vi "runtest empty test execution settings.vi"() -> (0 "empty Test Execution Settings":T1={"Quick Mode (T)"=FALSE, "Seq Count"=0, "Step Info"="", "Instruments on Station"=[], "LANGUAGE"="English", "Files Found?"=FALSE, "Step Number"=1} {"Step Number" min=1 step=1})   [LabVIEW 2011]
uses:
  tests/Test Execution Settings.ctl
  server/database/Stations/Instruments/Instrument Record.ctl
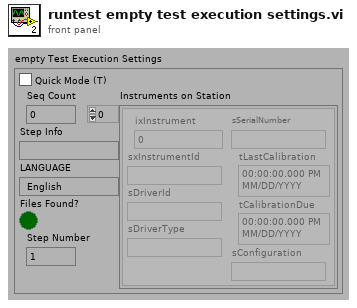
[diagram p1: front panel]
types:
  T1 = typedef "Test Execution Settings.ctl" = cluster{"Quick Mode (T)":bool, "Seq Count":i32, "Step Info":string, "Instruments on Station":T2[], "LANGUAGE":string, "Files Found?":bool, "Step Number":i32}
  T2 = typedef "Instrument Record.ctl" = cluster{"ixInstrument":i32, "sxInstrumentId":string, "sDriverId":string, "sDriverType":string, "sSerialNumber":string, "tLastCalibration":timestamp, "tCalibrationDue":timestamp, "sConfiguration":string}
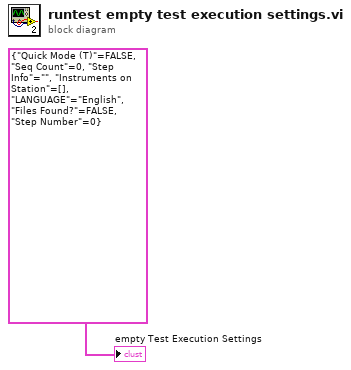
[diagram p0: block diagram]
diagram:
  "empty Test Execution Settings" <- T1 {"Quick Mode (T)"=FALSE, "Seq Count"=0, "Step Info"="", "Instruments on Station"=[], "LANGUAGE"="English", "Files Found?"=FALSE, "Step Number"=0} ("Test Execution Settings")
